vi "ConveyorControl.vi"(10 "ConveyorAct":refnum<vi>, 11 "Station Action in":refnum<class "Station Action.lvclass">) -> (3 "Station Action Out":refnum<class "Station Action.lvclass">)   [LabVIEW 2019]
uses:
  Ctrl/Conveyor Action.ctl
  Station Action.lvclass
  Ctrl/Auto Inspection Data Name.ctl
  FlowCtrl Class/Ctrl/Auto Inspection_IN Name.ctl
  FlowCtrl Class/Ctrl/Auto Inspection_Out Name.ctl
  Ctrl/Auto Inspection Main UI Ref.ctl
  Function/Main UI/Glb/Main_UI Gb.vi
  LLB/Commonly VI.lvlib
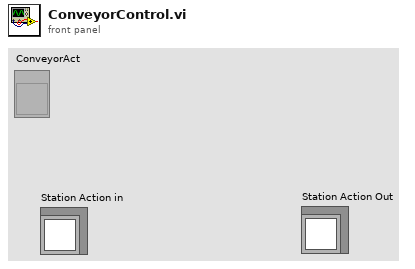
[diagram p1: front panel]
types:
  T1 = typedef "Conveyor Action.ctl" = enum16{"CheckWorkStationStatus", "Request Item In", "Check Product Ready In", "Wait Item In", "Check SlowSignal And Slow", "Check Arrive", "Rise Tray", "FixTray", "Imform Robot", "Wait Robot Imform", "DropTray Imform Out", "Wait Request ", "Flow Out"}
  T2 = cluster{"AutoRunFlg":refnum<vi>, "Action Finish Flg":refnum<vi>, "Remaining Action":refnum<vi>, "Btn_AutoRun":refnum<vi>, "Manual Flg":refnum<vi>, "Sub Process Error":refnum<vi>}
  T3 = typedef "Auto Inspection Data Name.ctl" = enum16{"LocalRun", "ItemSN(TimeCode)", "CurrentAction", "Error"}
  T4 = typedef "Auto Inspection_IN Name.ctl" = enum16{"ItemInWorkPos", "ItemReadyIn", "ItemInSensor", "StopUpSensor", "SlowSensor", "TrayUp", "Fix", "Release fix", "TrayDown", "NextRequest", "StopDown", "ConveyorOut"}
  T5 = typedef "Auto Inspection_Out Name.ctl" = enum16{"RequestItem", "ConeyorMotor", "WorkPosStopper", "SlowConveyor", "Rise", "Fix", "ImformOut"}
  T6 = typedef "Auto Inspection Main UI Ref.ctl" = cluster{"LineScan arrive":refnum<vi>, "LineScanfinish":refnum<vi>, "AI arrive":refnum<vi>, "AI finish":refnum<vi>, "NG Pick arrive":refnum<vi>, "NG Pick finish":refnum<vi>}
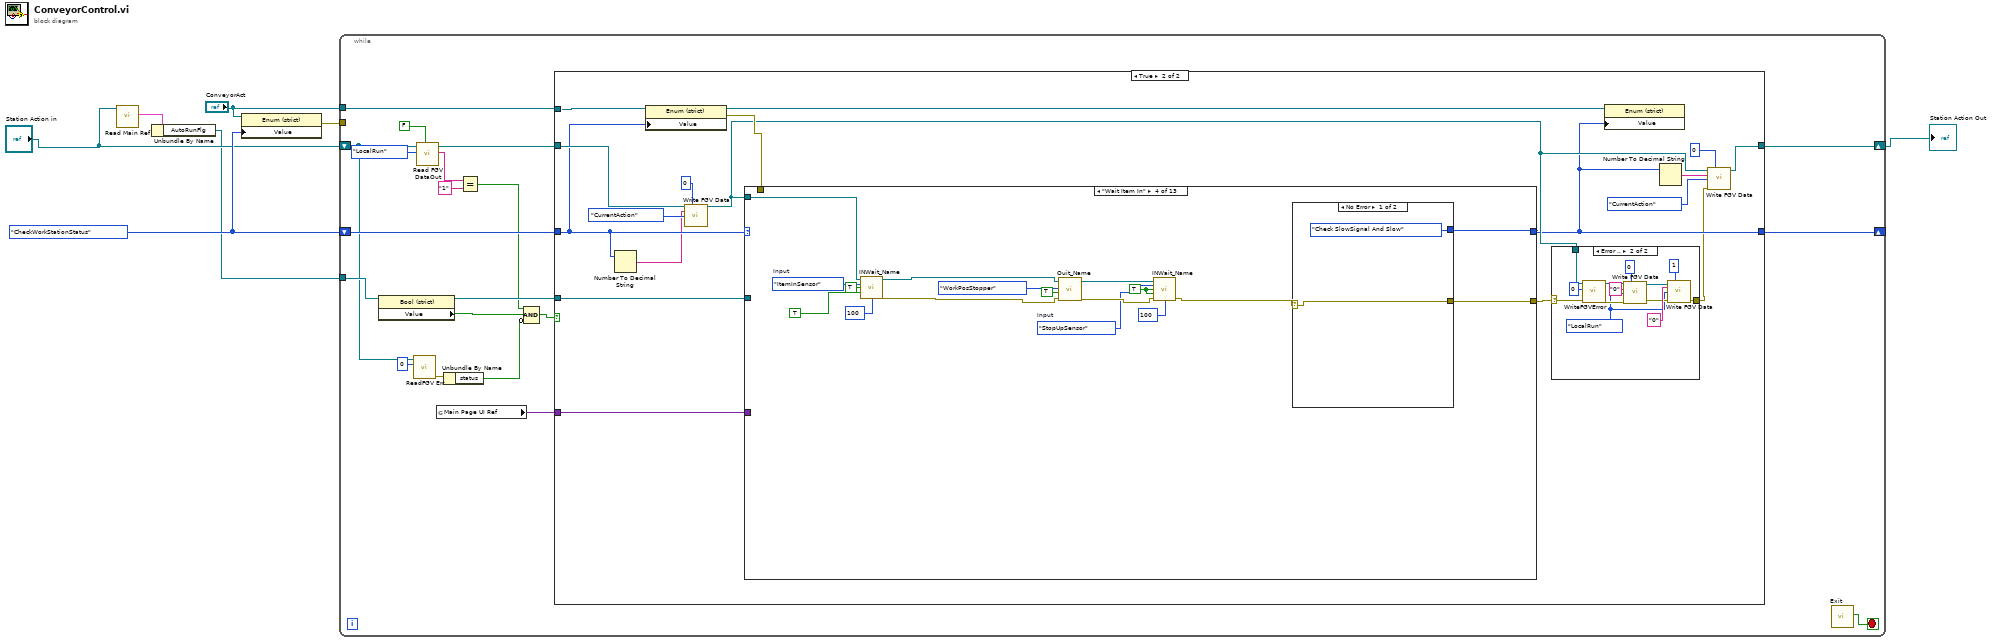
[diagram p0: block diagram]
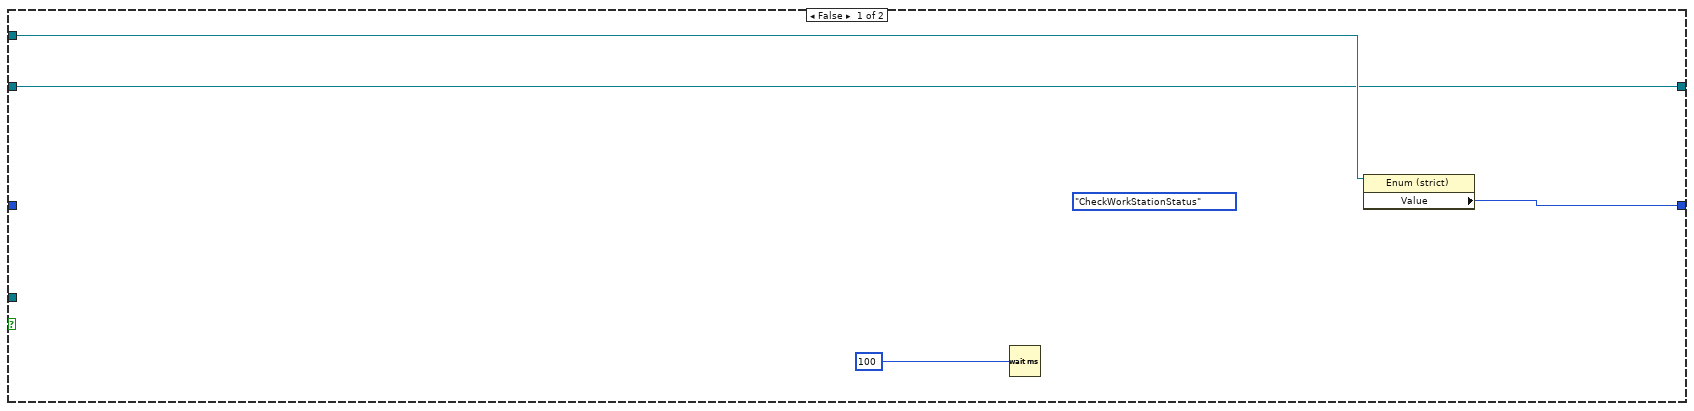
[diagram p2: hidden frame]
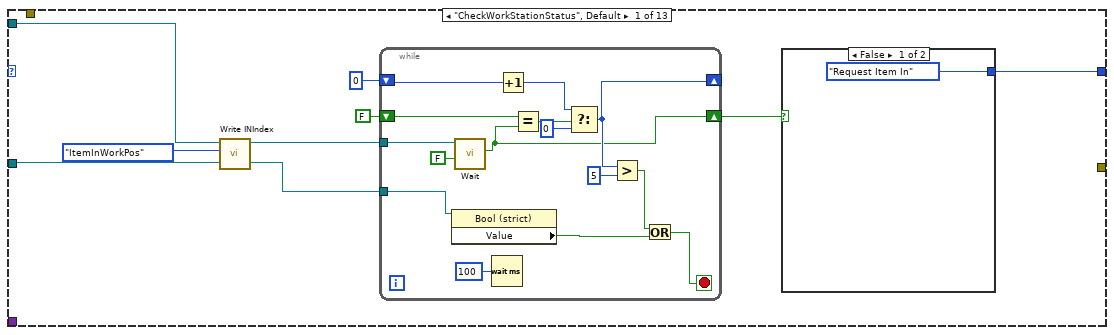
[diagram p4: hidden frame]
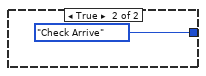
[diagram p5: hidden frame]
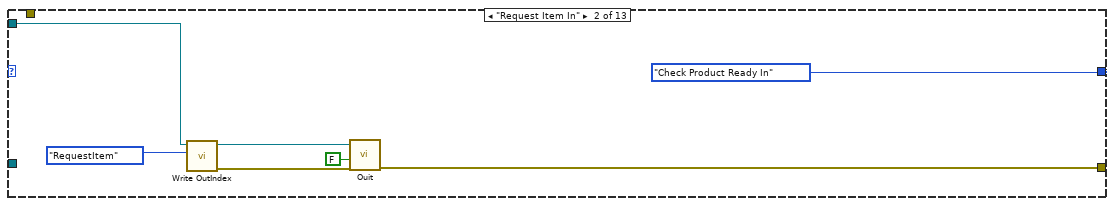
[diagram p6: hidden frame]
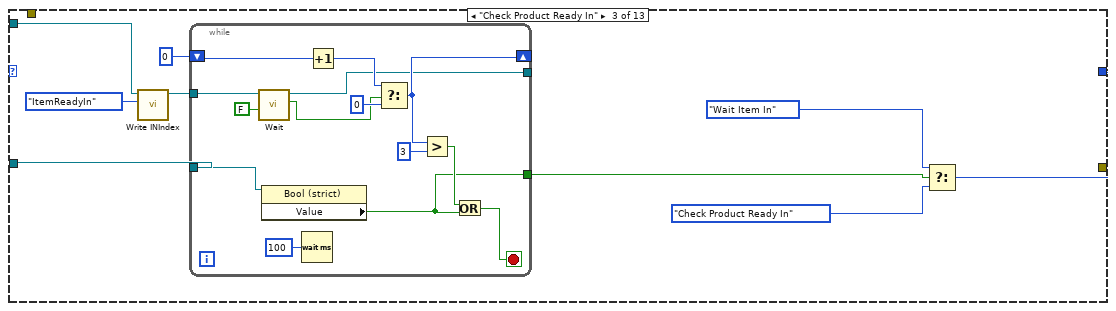
[diagram p7: hidden frame]
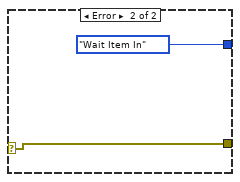
[diagram p8: hidden frame]
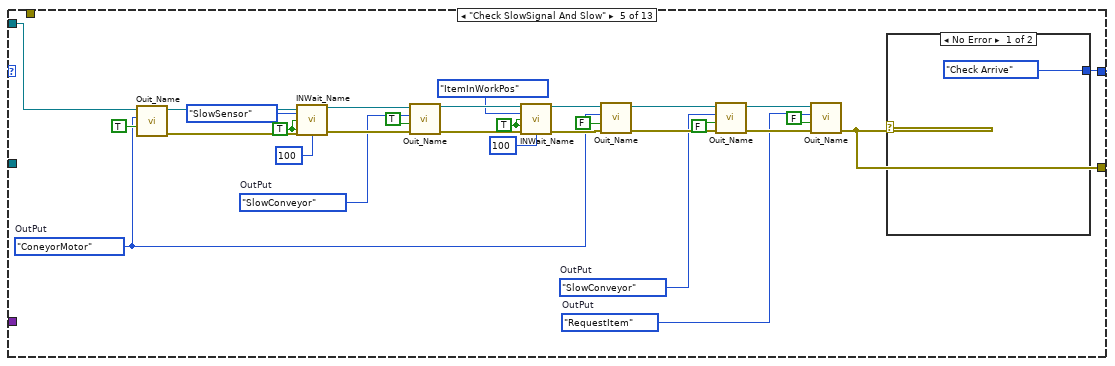
[diagram p9: hidden frame]
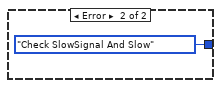
[diagram p10: hidden frame]
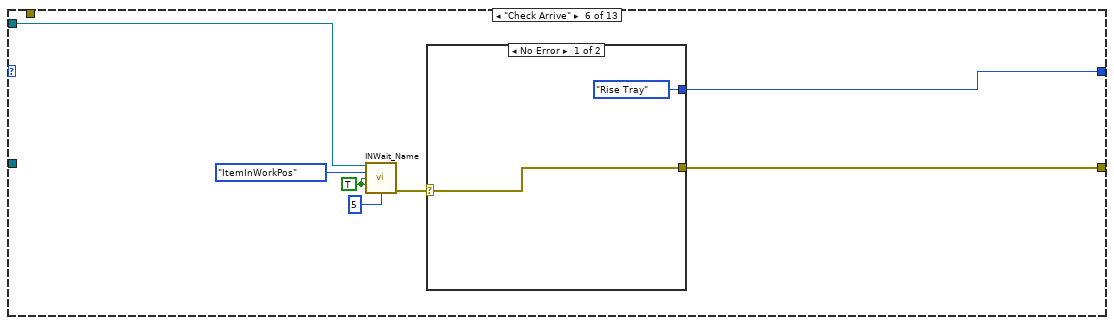
[diagram p11: hidden frame]
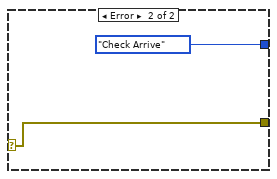
[diagram p12: hidden frame]
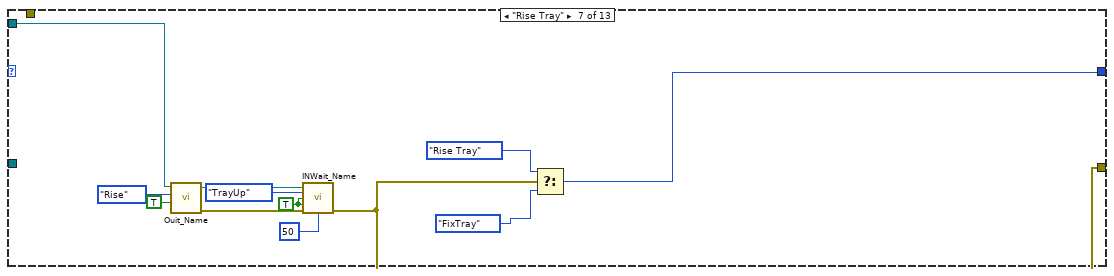
[diagram p13: hidden frame]
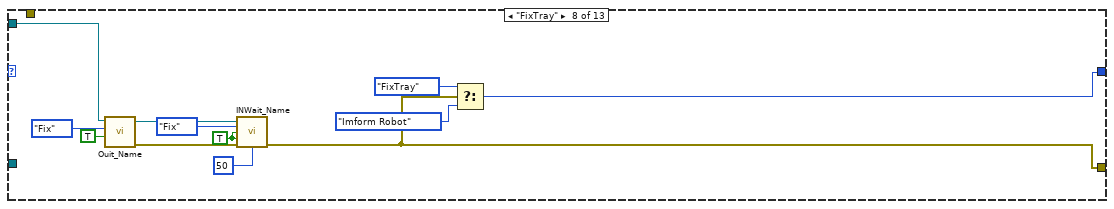
[diagram p14: hidden frame]
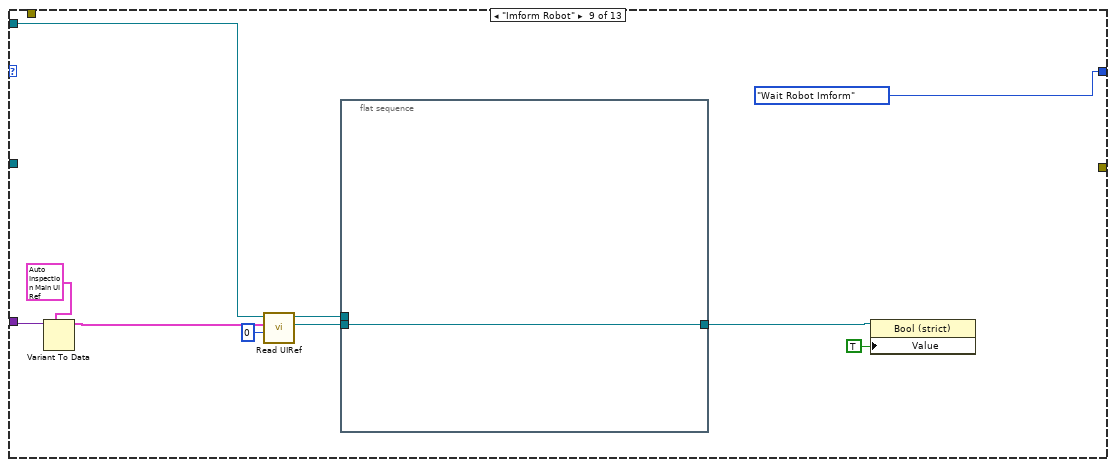
[diagram p15: hidden frame]
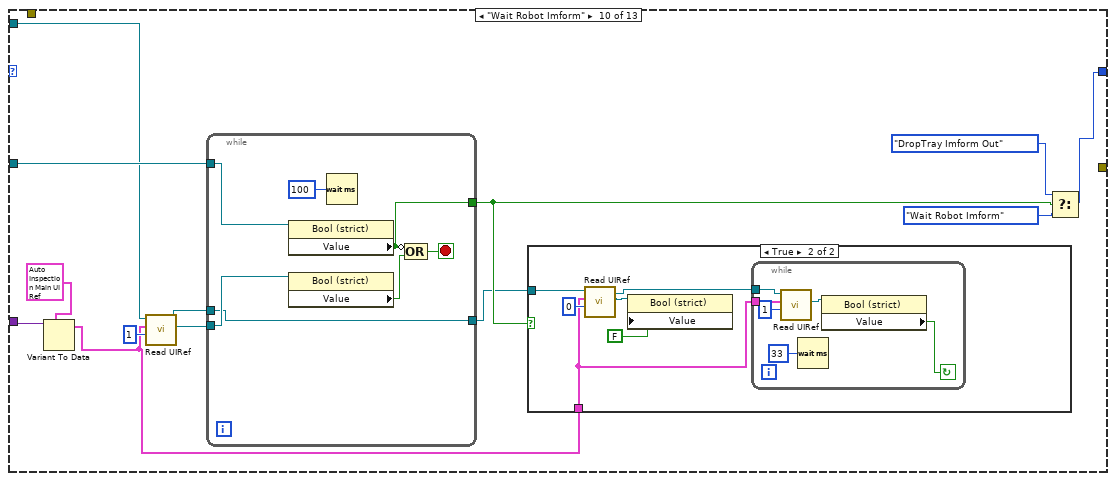
[diagram p16: hidden frame]
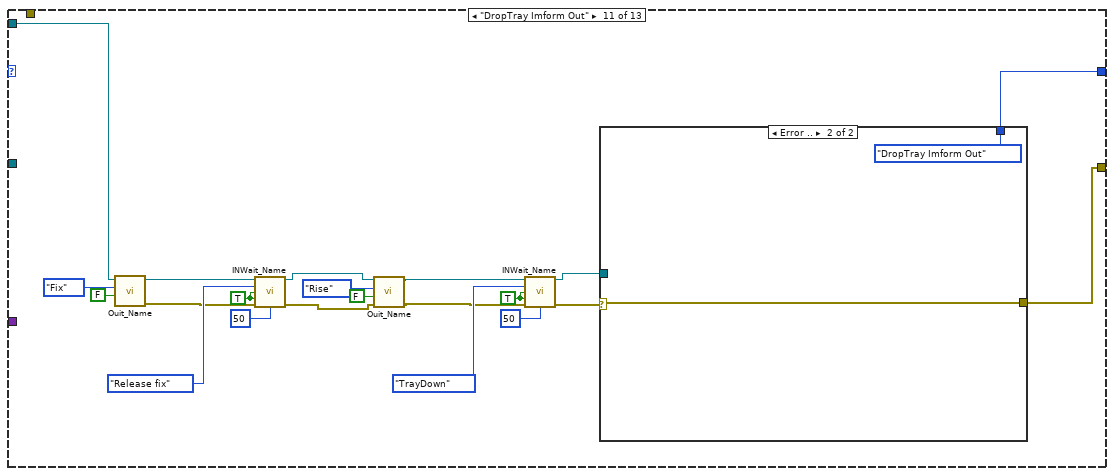
[diagram p18: hidden frame]
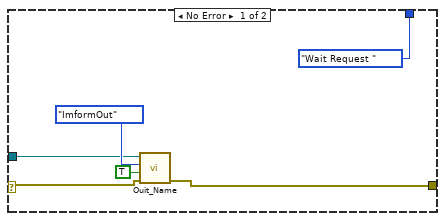
[diagram p19: hidden frame]
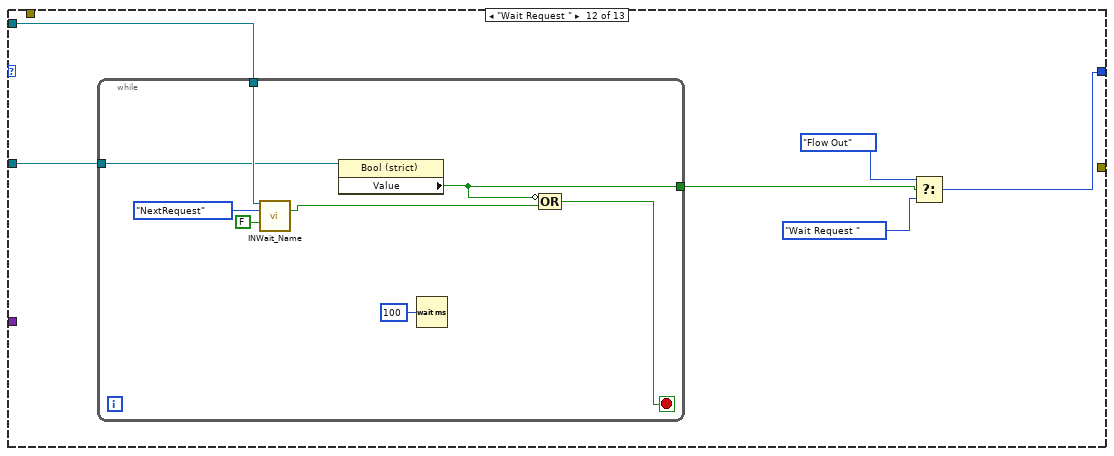
[diagram p20: hidden frame]
diagram:
  w5 = Conveyor_Action."CheckWorkStationStatus"
  n1 = call-dynamic "Read Main Ref.vi"("Main Process Class in"="Station Action in") -> ("Main Ref"=w2:T2)  [unwired: 8 in, 2 out]
  n2 = Unbundle By Name(w2) -> ("AutoRunFlg"=w1:refnum<vi>)
  n3 = property class="Enum (strict)"(reference="ConveyorAct", "Value"=w5) -> (error out=w6:errorcluster)  [unwired: 1 in, 1 out]
  n4 = while {
    shift-right: [w22] -> _
    shift-left: w5 -> [w24]
    tunnel: w1 -> [w27]
    shift-right: [w14] -> w4
    shift-left: "Station Action in" -> [w15]
    tunnel: "ConveyorAct" -> [w20]
    tunnel: w6 -> [_]
    stop <- w19 stop-if-true
    n5 = property class="Bool (strict)"(reference=w27) -> (reference out=w23:refnum<vi>, "Value"=w26:bool)  [unwired: 1 in, 1 out]
    n6 = call-dynamic "ReadFGV Err.vi"("0Cv/1ST"=0, "Station Action in"=w15) -> ("error out"=w18:errorcluster)  [unwired: 8 in, 1 out]
    n7 = call-dynamic "Read FGV DataOut.vi"("TSt/FConveyor"=FALSE, "Data"=Auto_Inspection_Data_Name."LocalRun", "Station Action in"=w15) -> ("DataOut"=w10:string, "Station Action out"=w13:refnum<class "Station Action.lvclass">)  [unwired: 6 in, 1 out]
    n8 = global read "Main_UI Gb.vi" "Main Page UI Ref"() -> (w21:variant)
    n9 = Unbundle By Name(w18) -> ("status"=w17:bool)
    n10 = Equal?(x=w10, y="1") -> (x = y?=w8:bool)
    n11 = Compound Arithmetic op=AND(w8, w26, invert w17) -> (w25:bool)
    n12 = case shown="True" w25 {
      tunnel: w24 -> [_ w41]
      tunnel: w23 -> [_ w49]
      tunnel: [w31 w35] -> w22
      tunnel: w13 -> [w28 w44]
      tunnel: w21 -> [_ w48]
      tunnel: w20 -> [w30 w47]
      tunnel: [w28 w33] -> w14
      frame False {
        (unwired) Conveyor_Action."CheckWorkStationStatus" ("Value")
        n13 = Wait (ms)(milliseconds to wait=u32 100) -> ()  [unwired: 1 out]
        n14 = property class="Enum (strict)"(reference=w30) -> ("Value"=w31:T1)  [unwired: 1 in, 2 out]
      }
      frame True {
        n15 = Number To Decimal String(number=w41) -> (decimal integer string=w40:string)  [unwired: 1 in]
        n16 = property class="Enum (strict)"(reference=w47, "Value"=w41) -> (reference out=w46:refnum<vi>, error out=w45:errorcluster)  [unwired: 1 in]
        n17 = call-dynamic "Write FGV Data.vi"("Station Action in"=w44, "0Cv/1St"=0, "DataIn"=w40, "Data"=Auto_Inspection_Data_Name."CurrentAction") -> ("Station Action out"=w36:refnum<class "Station Action.lvclass">)  [unwired: 10 in, 1 out]
        n18 = case shown="\"Wait Item In\"" w41 {
          tunnel: w49 -> [w69 _ w103 _ _ _ _ _ _ w228 _ w283 _]
          tunnel: [w67 Conveyor_Action."Check Product Ready In" w96 w131 w140 w172 w184 w196 Conveyor_Action."Wait Robot Imform" ("t") w226 w250 w279 w294] -> w35
          tunnel: w36 -> [w66 w94 w102 w130 w146 w176 w192 w199 w212 w223 w268 w284 w313]
          tunnel: [_ w89 _ w132 w141 w173 w183 w198 _ _ w252 _ w293] -> w34
          tunnel: w48 -> [_ _ _ _ _ _ _ _ w214 w229 _ _ _]
          tunnel: w45 -> [_ _ _ _ _ _ _ _ _ _ _ _ _]
          frame "CheckWorkStationStatus", Default {
            n19 = call-dynamic "Write INIndex.vi"("INIndex"=Auto_Inspection_IN_Name."ItemInWorkPos", "Station Action in"=w66) -> ("Station Action out"=w65:refnum<class "Station Action.lvclass">)  [unwired: 8 in, 1 out]
            n20 = while {
              shift-right: [w75] -> w68
              shift-left: FALSE -> [w88]
              shift-right: [w81] -> _
              shift-left: 0 -> [w86]
              tunnel: w69 -> [w82]
              tunnel: w65 -> [w76]
              stop <- w78 stop-if-true
              n21 = property class="Bool (strict)"(reference=w82) -> ("Value"=w77:bool)  [unwired: 1 in, 2 out]
              n22 = call-dynamic "Wait.vi"("Wait?"=FALSE, "FlowCtrl in"=w76) -> ("StatusOut"=w75:bool)  [unwired: 6 in, 3 out]
              n23 = Wait (ms)(milliseconds to wait=u32 100) -> ()  [unwired: 1 out]
              n24 = Increment(x=w86) -> (x+1=w85:i32)
              n25 = Equal?(x=w88, y=w75) -> (x = y?=w84:bool)
              n26 = Select(t=w85, s=w84, f=0) -> (s? t:f=w81:i32)
              n27 = Greater?(x=w81, y=5) -> (0:w79:bool)
              n28 = Or(x=w79, y=w77) -> (x .or. y?=w78:bool)
            }
            n29 = case shown="False" w68 {
              tunnel: [Conveyor_Action."Request Item In" Conveyor_Action."Check Arrive"] -> w67
              frame False {
              }
              frame True {
              }
            }
          }
          frame "Request Item In" {
            n30 = call-dynamic "Write OutIndex.vi"("OutIndex"=Auto_Inspection_Out_Name."RequestItem", "Station Action in"=w94) -> ("error out"=w90:errorcluster, "Station Action out"=w93:refnum<class "Station Action.lvclass">)  [unwired: 8 in]
            n31 = call-dynamic "Ouit.vi"("error in (no error)"=w90, "BL"=FALSE, "FlowCtrl in"=w93) -> ("error out"=w89:errorcluster)  [unwired: 7 in, 1 out]
          }
          frame "Check Product Ready In" {
            n32 = call-dynamic "Write INIndex.vi"("INIndex"=Auto_Inspection_IN_Name."ItemReadyIn", "Station Action in"=w102) -> ("Station Action out"=w100:refnum<class "Station Action.lvclass">)  [unwired: 8 in, 1 out]
            n33 = while {
              shift-right: [w113] -> _
              shift-left: 0 -> [w117]
              tunnel: w103 -> [w114]
              tunnel: [w109] -> w99
              tunnel: w100 -> [w107]
              tunnel: [w105] -> _
              stop <- w110 stop-if-true
              n34 = call-dynamic "Wait.vi"("Wait?"=FALSE, "FlowCtrl in"=w107) -> ("StatusOut"=w106:bool, "FlowCtrl out"=w105:refnum<class "Station Action.lvclass">)  [unwired: 6 in, 2 out]
              n35 = property class="Bool (strict)"(reference=w114) -> ("Value"=w109:bool)  [unwired: 1 in, 2 out]
              n36 = Wait (ms)(milliseconds to wait=u32 100) -> ()  [unwired: 1 out]
              n37 = Increment(x=w117) -> (x+1=w116:i32)
              n38 = Select(t=w116, s=w106, f=0) -> (s? t:f=w113:i32)
              n39 = Greater?(x=w113, y=3) -> (0:w111:bool)
              n40 = Or(x=w111, y=w109) -> (x .or. y?=w110:bool)
            }
            n41 = Select(t=Conveyor_Action."Wait Item In", s=w99, f=Conveyor_Action."Check Product Ready In") -> (s? t:f=w96:T1)
          }
          frame "Wait Item In" {
            w120 = TRUE ("Status")
            w121 = Auto_Inspection_IN_Name."StopUpSensor"  # Input
            w134 = Auto_Inspection_IN_Name."ItemInSensor"  # Input
            n42 = call "INWait_Name.vi"("FlowCtrl in"=w130, "Input"=w134, "Status"=TRUE, "Wait?"=TRUE, "time(0.1)"=100) -> ("FlowCtrl out"=w128:refnum<class "Station Action.lvclass">, "error out"=w126:errorcluster)  [unwired: 7 in, 2 out]
            n43 = call "Ouit_Name.vi"("error in (no error)"=w126, "BL"=TRUE, "OutPut"=Auto_Inspection_Out_Name."WorkPosStopper", "FlowCtrl in"=w128) -> ("error out"=w122:errorcluster, "FlowCtrl out"=w123:refnum<class "Station Action.lvclass">)  [unwired: 6 in]
            n44 = call "INWait_Name.vi"("FlowCtrl in"=w123, "Input"=w121, "Status"=w120, "Wait?"=w120, "error in (no error)"=w122, "time(0.1)"=100) -> ("error out"=w119:errorcluster)  [unwired: 6 in, 3 out]
            n45 = case shown="No Error" w119 {
              selector: w119 -> [w137 w139]
              tunnel: [w137 w139] -> w132
              tunnel: [Conveyor_Action."Check SlowSignal And Slow" Conveyor_Action."Wait Item In"] -> w131
              frame No Error {
              }
              frame Error {
              }
            }
          }
          frame "Check SlowSignal And Slow" {
            w142 = TRUE ("Wait?")
            w143 = TRUE ("Wait?")
            w149 = Auto_Inspection_Out_Name."RequestItem"  # OutPut
            w151 = Auto_Inspection_Out_Name."SlowConveyor"  # OutPut
            w145 = Auto_Inspection_Out_Name."ConeyorMotor"  # OutPut
            w156 = Auto_Inspection_Out_Name."SlowConveyor"  # OutPut
            n46 = call "Ouit_Name.vi"("BL"=TRUE, "OutPut"=w145, "FlowCtrl in"=w146) -> ("error out"=w144:errorcluster, "FlowCtrl out"=w147:refnum<class "Station Action.lvclass">)  [unwired: 7 in]
            n47 = call "INWait_Name.vi"("FlowCtrl in"=w147, "Input"=Auto_Inspection_IN_Name."SlowSensor", "Status"=w143, "Wait?"=w143, "error in (no error)"=w144, "time(0.1)"=100) -> ("FlowCtrl out"=w161:refnum<class "Station Action.lvclass">, "error out"=w160:errorcluster)  [unwired: 6 in, 2 out]
            n48 = call "Ouit_Name.vi"("error in (no error)"=w160, "BL"=TRUE, "OutPut"=w156, "FlowCtrl in"=w161) -> ("error out"=w162:errorcluster, "FlowCtrl out"=w163:refnum<class "Station Action.lvclass">)  [unwired: 6 in]
            n49 = call "INWait_Name.vi"("FlowCtrl in"=w163, "Input"=Auto_Inspection_IN_Name."ItemInWorkPos", "Status"=w142, "Wait?"=w142, "error in (no error)"=w162, "time(0.1)"=100) -> ("FlowCtrl out"=w165:refnum<class "Station Action.lvclass">, "error out"=w164:errorcluster)  [unwired: 6 in, 2 out]
            n50 = call "Ouit_Name.vi"("error in (no error)"=w164, "BL"=FALSE, "OutPut"=w145, "FlowCtrl in"=w165) -> ("error out"=w166:errorcluster, "FlowCtrl out"=w167:refnum<class "Station Action.lvclass">)  [unwired: 6 in]
            n51 = call "Ouit_Name.vi"("error in (no error)"=w166, "BL"=FALSE, "OutPut"=w151, "FlowCtrl in"=w167) -> ("error out"=w168:errorcluster, "FlowCtrl out"=w169:refnum<class "Station Action.lvclass">)  [unwired: 6 in]
            n52 = call "Ouit_Name.vi"("error in (no error)"=w168, "BL"=FALSE, "OutPut"=w149, "FlowCtrl in"=w169) -> ("error out"=w141:errorcluster)  [unwired: 6 in, 1 out]
            n53 = case shown="No Error" w141 {
              tunnel: [Conveyor_Action."Check Arrive" Conveyor_Action."Check SlowSignal And Slow"] -> w140
              frame No Error {
              }
              frame Error {
              }
            }
          }
          frame "Check Arrive" {
            w178 = TRUE ("Wait?")
            n54 = call "INWait_Name.vi"("FlowCtrl in"=w176, "Input"=Auto_Inspection_IN_Name."ItemInWorkPos", "Status"=w178, "Wait?"=w178, "time(0.1)"=5) -> ("error out"=w174:errorcluster)  [unwired: 7 in, 3 out]
            n55 = case shown="No Error" w174 {
              selector: w174 -> [w180 w181]
              tunnel: [w180 w181] -> w173
              tunnel: [Conveyor_Action."Rise Tray" Conveyor_Action."Check Arrive"] -> w172
              frame No Error {
              }
              frame Error {
              }
            }
          }
          frame "Rise Tray" {
            w191 = TRUE ("Wait?")
            n56 = call "Ouit_Name.vi"("BL"=TRUE, "OutPut"=Auto_Inspection_Out_Name."Rise", "FlowCtrl in"=w192) -> ("error out"=w188:errorcluster, "FlowCtrl out"=w187:refnum<class "Station Action.lvclass">)  [unwired: 7 in]
            n57 = call "INWait_Name.vi"("FlowCtrl in"=w187, "Input"=Auto_Inspection_IN_Name."TrayUp", "Status"=w191, "Wait?"=w191, "error in (no error)"=w188, "time(0.1)"=50) -> ("error out"=w183:errorcluster)  [unwired: 6 in, 3 out]
            n58 = Select(t=Conveyor_Action."Rise Tray", s=w183, f=Conveyor_Action."FixTray") -> (s? t:f=w184:T1)
          }
          frame "FixTray" {
            w203 = TRUE ("Wait?")
            n59 = call "Ouit_Name.vi"("BL"=TRUE, "OutPut"=Auto_Inspection_Out_Name."Fix", "FlowCtrl in"=w199) -> ("error out"=w206:errorcluster, "FlowCtrl out"=w205:refnum<class "Station Action.lvclass">)  [unwired: 7 in]
            n60 = call "INWait_Name.vi"("FlowCtrl in"=w205, "Input"=Auto_Inspection_IN_Name."Fix", "Status"=w203, "Wait?"=w203, "error in (no error)"=w206, "time(0.1)"=50) -> ("error out"=w198:errorcluster)  [unwired: 6 in, 3 out]
            n61 = Select(t=Conveyor_Action."FixTray", s=w198, f=Conveyor_Action."Imform Robot") -> (s? t:f=w196:T1)
          }
          frame "Imform Robot" {
            n62 = Variant To Data(type=T6 {"LineScan arrive"=refnum, "LineScanfinish"=refnum, "AI arrive"=refnum, "AI finish"=refnum, "NG Pick arrive"=refnum, "NG Pick finish"=refnum} ("UI Ref"), Variant=w214) -> (data=w211:T6)  [unwired: 1 in, 1 out]
            n63 = call-dynamic "Read UIRef.vi"("0Arrive/1Finish"=0, "UI Ref"=w211, "Station Action in"=w212) -> ("RefOut"=w208:refnum<vi>, "Station Action out"=w207:refnum<class "Station Action.lvclass">)  [unwired: 6 in, 1 out]
            n64 = flat-sequence {
              tunnel: [w217] -> w209
              tunnel: w208 -> [w217]
              tunnel: w207 -> [_]
              frame #0 {
              }
            }
            n65 = property class="Bool (strict)"(reference=w209, "Value"=TRUE) -> ()  [unwired: 1 in, 2 out]
          }
          frame "Wait Robot Imform" {
            n66 = Variant To Data(type=T6 {"LineScan arrive"=refnum, "LineScanfinish"=refnum, "AI arrive"=refnum, "AI finish"=refnum, "NG Pick arrive"=refnum, "NG Pick finish"=refnum} ("UI Ref"), Variant=w229) -> (data=w218:T6)  [unwired: 1 in, 1 out]
            n67 = call-dynamic "Read UIRef.vi"("0Arrive/1Finish"=1, "UI Ref"=w218, "Station Action in"=w223) -> ("RefOut"=w222:refnum<vi>, "Station Action out"=w221:refnum<class "Station Action.lvclass">)  [unwired: 6 in, 1 out]
            n68 = while {
              tunnel: w222 -> [w249]
              tunnel: w228 -> [w248]
              tunnel: [w244] -> w220
              tunnel: [w243] -> w219
              tunnel: w221 -> [w243]
              stop <- w245 stop-if-true
              n69 = property class="Bool (strict)"(reference=w248) -> ("Value"=w244:bool)  [unwired: 1 in, 2 out]
              n70 = property class="Bool (strict)"(reference=w249) -> ("Value"=w246:bool)  [unwired: 1 in, 2 out]
              n71 = Wait (ms)(milliseconds to wait=u32 100) -> ()  [unwired: 1 out]
              n72 = Compound Arithmetic op=OR(invert w244, w246) -> (w245:bool)
            }
            n73 = case shown="True" w220 {
              tunnel: w219 -> [_ w233]
              tunnel: w218 -> [_ w231]
              frame False {
              }
              frame True {
                n74 = call-dynamic "Read UIRef.vi"("0Arrive/1Finish"=0, "UI Ref"=w231, "Station Action in"=w233) -> ("RefOut"=w236:refnum<vi>, "Station Action out"=w232:refnum<class "Station Action.lvclass">)  [unwired: 6 in, 1 out]
                n75 = property class="Bool (strict)"(reference=w236, "Value"=FALSE) -> ()  [unwired: 1 in, 2 out]
                n76 = while {
                  tunnel: w232 -> [w242]
                  tunnel: w231 -> [w241]
                  stop <- w237 continue-if-true
                  n77 = call-dynamic "Read UIRef.vi"("0Arrive/1Finish"=1, "UI Ref"=w241, "Station Action in"=w242) -> ("RefOut"=w238:refnum<vi>)  [unwired: 6 in, 2 out]
                  n78 = Wait (ms)(milliseconds to wait=u32 33) -> ()  [unwired: 1 out]
                  n79 = property class="Bool (strict)"(reference=w238) -> ("Value"=w237:bool)  [unwired: 1 in, 2 out]
                }
              }
            }
            n80 = Select(t=Conveyor_Action."DropTray Imform Out", s=w220, f=Conveyor_Action."Wait Robot Imform" ("t")) -> (s? t:f=w226:T1)
          }
          frame "DropTray Imform Out" {
            w256 = TRUE ("Wait?")
            w267 = TRUE ("Wait?")
            n81 = call "Ouit_Name.vi"("BL"=FALSE, "OutPut"=Auto_Inspection_Out_Name."Fix", "FlowCtrl in"=w268) -> ("error out"=w263:errorcluster, "FlowCtrl out"=w264:refnum<class "Station Action.lvclass">)  [unwired: 7 in]
            n82 = call "INWait_Name.vi"("FlowCtrl in"=w264, "Input"=Auto_Inspection_IN_Name."Release fix", "Status"=w267, "Wait?"=w267, "error in (no error)"=w263, "time(0.1)"=50) -> ("FlowCtrl out"=w260:refnum<class "Station Action.lvclass">, "error out"=w259:errorcluster)  [unwired: 6 in, 2 out]
            n83 = call "Ouit_Name.vi"("error in (no error)"=w259, "BL"=FALSE, "OutPut"=Auto_Inspection_Out_Name."Rise", "FlowCtrl in"=w260) -> ("error out"=w254:errorcluster, "FlowCtrl out"=w255:refnum<class "Station Action.lvclass">)  [unwired: 6 in]
            n84 = call "INWait_Name.vi"("FlowCtrl in"=w255, "Input"=Auto_Inspection_IN_Name."TrayDown", "Status"=w256, "Wait?"=w256, "error in (no error)"=w254, "time(0.1)"=50) -> ("FlowCtrl out"=w251:refnum<class "Station Action.lvclass">, "error out"=w253:errorcluster)  [unwired: 6 in, 2 out]
            n85 = case shown="Error .." w253 {
              selector: w253 -> [w274 w277]
              tunnel: [w273 w277] -> w252
              tunnel: w251 -> [w272 _]
              tunnel: [Conveyor_Action."Wait Request " ("t") Conveyor_Action."DropTray Imform Out" ("t")] -> w250
              frame No Error {
                n86 = call "Ouit_Name.vi"("error in (no error)"=w274, "BL"=TRUE, "OutPut"=Auto_Inspection_Out_Name."ImformOut", "FlowCtrl in"=w272) -> ("error out"=w273:errorcluster)  [unwired: 6 in, 1 out]
              }
              frame Error {
              }
            }
          }
          frame "Wait Request " {
            n87 = while {
              tunnel: w284 -> [w290]
              tunnel: w283 -> [w289]
              tunnel: [w285] -> w282
              stop <- w287 stop-if-true
              n88 = call "INWait_Name.vi"("FlowCtrl in"=w290, "Input"=Auto_Inspection_IN_Name."NextRequest", "Wait?"=FALSE) -> ("StatusOut"=w288:bool)  [unwired: 9 in, 3 out]
              n89 = property class="Bool (strict)"(reference=w289) -> ("Value"=w285:bool)  [unwired: 1 in, 2 out]
              n90 = Wait (ms)(milliseconds to wait=u32 100) -> ()  [unwired: 1 out]
              n91 = Compound Arithmetic op=OR(invert w285, w288) -> (w287:bool)
            }
            n92 = Select(t=Conveyor_Action."Flow Out", s=w282, f=Conveyor_Action."Wait Request " ("t")) -> (s? t:f=w279:T1)
          }
          frame "Flow Out" {
            w295 = Auto_Inspection_IN_Name."ConveyorOut" ("Input")
            n93 = call "Ouit_Name.vi"("BL"=FALSE, "OutPut"=Auto_Inspection_Out_Name."WorkPosStopper", "FlowCtrl in"=w313) -> ("error out"=w309:errorcluster, "FlowCtrl out"=w308:refnum<class "Station Action.lvclass">)  [unwired: 7 in]
            n94 = call "INWait_Name.vi"("FlowCtrl in"=w308, "Input"=Auto_Inspection_IN_Name."StopDown", "Status"=TRUE, "Wait?"=TRUE, "error in (no error)"=w309, "time(0.1)"=100) -> ("FlowCtrl out"=w304:refnum<class "Station Action.lvclass">, "error out"=w303:errorcluster)  [unwired: 6 in, 2 out]
            n95 = call "Ouit_Name.vi"("error in (no error)"=w303, "BL"=TRUE, "OutPut"=Auto_Inspection_Out_Name."ConeyorMotor", "FlowCtrl in"=w304) -> ("error out"=w298:errorcluster, "FlowCtrl out"=w299:refnum<class "Station Action.lvclass">)  [unwired: 6 in]
            n96 = call "INWait_Name.vi"("FlowCtrl in"=w299, "Input"=w295, "Status"=TRUE, "Wait?"=TRUE, "error in (no error)"=w298, "time(0.1)"=100) -> ("FlowCtrl out"=w296:refnum<class "Station Action.lvclass">, "error out"=w297:errorcluster)  [unwired: 6 in, 2 out]
            n97 = case shown="No Error" w297 {
              selector: w297 -> [_ w332]
              tunnel: w296 -> [w320 _]
              tunnel: w295 -> [w319 _]
              tunnel: [Conveyor_Action."Request Item In" ("t") Conveyor_Action."Flow Out" ("t")] -> w294
              tunnel: [errorcluster {"status"=FALSE, "code"=0, "source"=""} ("error IO") w332] -> w293
              frame No Error {
                n98 = while {
                  tunnel: w320 -> [w330]
                  tunnel: w319 -> [w329]
                  shift-right: [w323] -> _
                  shift-left: 0 -> [w327]
                  stop <- w321 stop-if-true
                  n99 = call "INWait_Name.vi"("FlowCtrl in"=w330, "Input"=w329, "Wait?"=FALSE) -> ("StatusOut"=w324:bool)  [unwired: 9 in, 3 out]
                  n100 = Increment(x=w327) -> (x+1=w326:i32)
                  n101 = Wait (ms)(milliseconds to wait=u32 100) -> ()  [unwired: 1 out]
                  n102 = Select(t=0, s=w324, f=w326) -> (s? t:f=w323:i32)
                  n103 = Greater?(x=w323, y=5) -> (0:w321:bool)
                }
              }
              frame Error {
              }
            }
          }
        }
        n104 = case shown="Error .." w34 {
          selector: w34 -> [w50 w61]
          tunnel: w36 -> [_ w63]
          tunnel: [w50 w51] -> w32
          frame No Error {
          }
          frame Error {
            w52 = Auto_Inspection_Data_Name."LocalRun" ("Data")
            n105 = call-dynamic "WriteFGVError.vi"("error in (no error)"=w61, "0Cv/1St"=0, "Station Action in"=w63) -> ("error out"=w57:errorcluster, "Station Action out"=w59:refnum<class "Station Action.lvclass">)  [unwired: 7 in]
            n106 = call-dynamic "Write FGV Data.vi"("Station Action in"=w59, "0Cv/1St"=0, "DataIn"="0", "Data"=w52, "error in (no error)"=w57) -> ("Station Action out"=w54:refnum<class "Station Action.lvclass">, "error out"=w53:errorcluster)  [unwired: 9 in]
            n107 = call-dynamic "Write FGV Data.vi"("Station Action in"=w54, "0Cv/1St"=1, "DataIn"="0", "Data"=w52, "error in (no error)"=w53) -> ("error out"=w51:errorcluster)  [unwired: 9 in, 1 out]
          }
        }
        n108 = property class="Enum (strict)"(reference=w46, "Value"=w35) -> ()  [unwired: 1 in, 2 out]
        n109 = Number To Decimal String(number=w35) -> (decimal integer string=w39:string)  [unwired: 1 in]
        n110 = call-dynamic "Write FGV Data.vi"("Station Action in"=w36, "0Cv/1St"=0, "DataIn"=w39, "Data"=Auto_Inspection_Data_Name."CurrentAction", "error in (no error)"=w32) -> ("Station Action out"=w33:refnum<class "Station Action.lvclass">)  [unwired: 9 in, 1 out]
      }
    }
    n111 = call "Exit.vi"() -> ("ExitOut"=w19:bool)  [unwired: 11 in]
  }
  "Station Action Out" <- w4
